vi "PUT_req_PS.vi"(7 "Headers":string, 8 "error in":errorcluster, 9 "ContentType":string, 10 "Body":string, 11 "URL":string) -> (0 "error out":errorcluster, 3 "PUT Request":string)   [LabVIEW 2020, in "Request.lvclass"]
uses:
  Request.lvclass
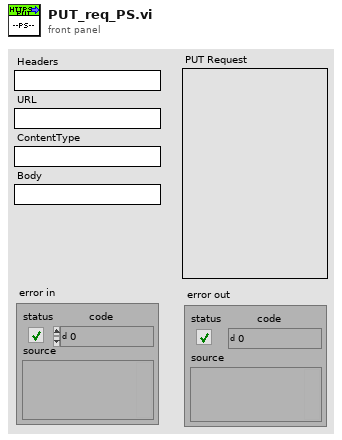
[diagram p1: front panel]
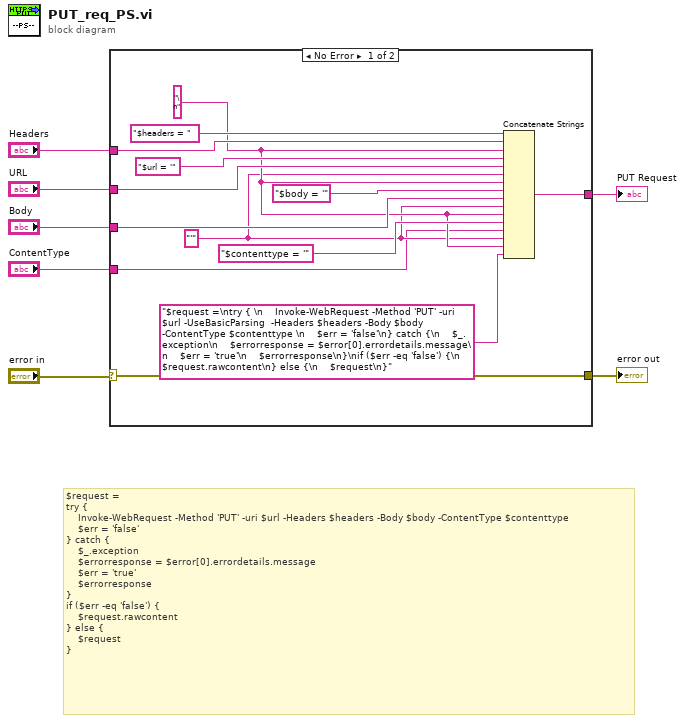
[diagram p0: block diagram]
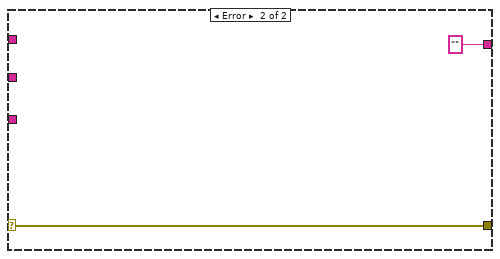
[diagram p2: hidden frame]
diagram:
  # "$request =\ntry { \n    Invoke-WebRequest -Method 'PUT' -uri $url -Headers $headers -Body $body -ContentType $contenttype \n    $err = 'false'\n} catch {\n    $_.exception\n    $errorresponse = $error[0].errordetails.message\n    $err = 'true'\n    $errorresponse\n}\nif ($err -eq 'false') {\n    $request.rawcontent\n} else {\n    $request\n}"
  n1 = case shown="No Error" "error in" {
    selector: "error in" -> [w15 w21]
    tunnel: "Headers" -> [w20 _]
    tunnel: "URL" -> [w17 _]
    tunnel: [w16 ""] -> w5
    tunnel: [w15 w21] -> w3
    tunnel: "Body" -> [w11 _]
    tunnel: "ContentType" -> [w8 _]
    frame No Error {
      w9 = "'" ("string")
      w10 = "\n"
      n2 = Concatenate Strings("$headers = ", w20, w10, "$url = '" ("string"), w17, w9, w10, "$body = '" ("string"), w11, w9, w10, "$contenttype = '" ("string"), w8, w9, w10, "$request =\ntry { \n    Invoke-WebRequest -Method 'PUT' -uri $url -UseBasicParsing  -Headers $headers -Body $body -ContentType $contenttype \n    $err = 'false'\n} catch {\n    $_.exception\n    $errorresponse = $error[0].errordetails.message\n    $err = 'true'\n    $errorresponse\n}\nif ($err -eq 'false') {\n    $request.rawcontent\n} else {\n    $request\n}" ("string")) -> (w16:string)
    }
    frame Error {
    }
  }
  "PUT Request" <- w5
  "error out" <- w3
